vi "Express VI - Filter.vi"() -> ()   [LabVIEW 2023]
doc: "This example shows some results of the use of the Filter Express VI."
uses:
  Instance           2 14Saved   Filter .vi
panel:
  out "Highpass Results":dynamicdata(graph)
  out "Bandpass Results":dynamicdata(graph)
  out "Lowpass Results":dynamicdata(graph)
  in  "Frequency":dbl(slide)=489.0 scale=1.0..5000.0
  in  "Stop":bool
  # "Overview: Demonstrates the use of the Filter Express VI.\nRequirements: LabVIEW Full Development System\nInstructions:\n1. Run the VI.\n2. Change the value of the Frequency for the original signal. See the results of the lowpass, bandpass and highpass filters on that signal as you increase the frequency.\n3. Click Stop to stop the VI.\n4. Open the block diagram and refer to the comments there."
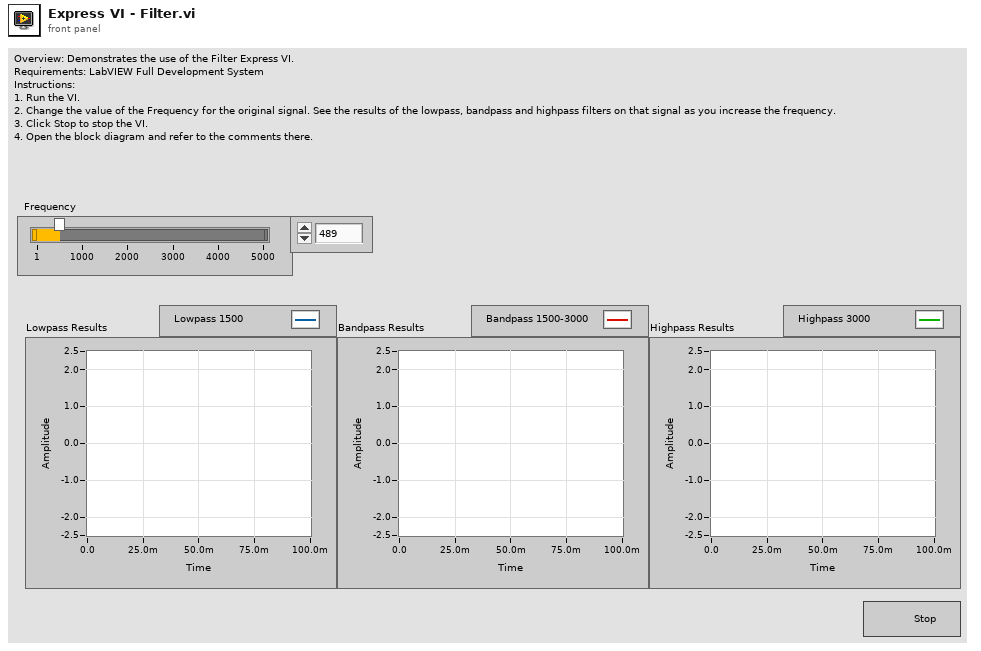
[diagram p1: front panel]
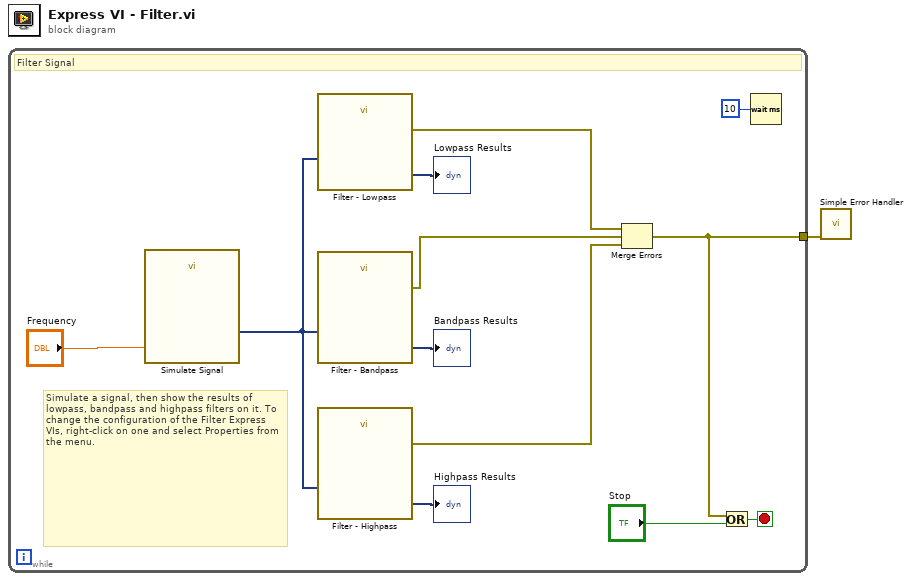
[diagram p0: block diagram]
diagram:
  n1 = while {
    tunnel: [w2] -> w1
    stop <- w3 stop-if-true
    # "Simulate a signal, then show the results of lowpass, bandpass and highpass filters on it. To change the configuration of the Filter Express VIs, right-click on one and select Properties from the menu."
    # "Filter Signal"
    n2 = call "Simulate Signal"("Frequency"="Frequency") -> ("Sine"=w8:dynamicdata)  [unwired: 13 in, 1 out]
    n3 = call "Filter - Lowpass"("Signal"=w8) -> ("error out"=w6:errorcluster, "Filtered Signal"=→"Lowpass Results":dynamicdata)  [unwired: 9 in]
    n4 = call "Filter - Bandpass"("Signal"=w8) -> ("error out"=w5:errorcluster, "Filtered Signal"=→"Bandpass Results":dynamicdata)  [unwired: 9 in]
    n5 = call "Filter - Highpass"("Signal"=w8) -> ("error out"=w4:errorcluster, "Filtered Signal"=→"Highpass Results":dynamicdata)  [unwired: 9 in]
    n6 = Merge Errors(w6, w5, w4) -> (w2:errorcluster)
    n7 = Or(x=w2, y="Stop") -> (x .or. y?=w3:bool)
    n8 = Wait (ms)(milliseconds to wait=u32 10) -> ()  [unwired: 1 out]
  }
  n9 = call <vilib>:"Simple Error Handler.vi"("error in (no error)"=w1) -> ()  [unwired: 4 in, 5 out]
